vi "Test Interpolation.vi"() -> ()   [LabVIEW 2012]
doc: "This example shows the operation of the 1D interpolation VI using three selectable test sets."
uses:
  <vilib>/gmath/NI_Gmath.lvlib
panel:
  in  "stop":bool
  in  "Tab Control":enum32{"Graph", "Data"}(tab)
  out "1D Interpolation Graph":cluster{"yi":dbl[], "ramp data":dbl[]}[](graph)
  out "Interpolated Data":dbl[][](array[numeric])
  out "Original Data":dbl[][](array[numeric])
  in  "Method":i32(ring)=2 items=["nearest", "linear", "spline", "cubic Hermite", "Lagrange"]
  in  "Data Sets":enum16{"Test Set 1", "Test Set 2", "Test Set 3"}(ring)
  # "The following example shows the operation of the 1D interpolation VI using three selectable test sets.\n\nInstructions:\n1) Run the VI\n2) Modify the Data Sets and interpolation Method, and view the results on both the Graph and Data tabs\n3) Stop the VI and look at the Block Diagram for more information"
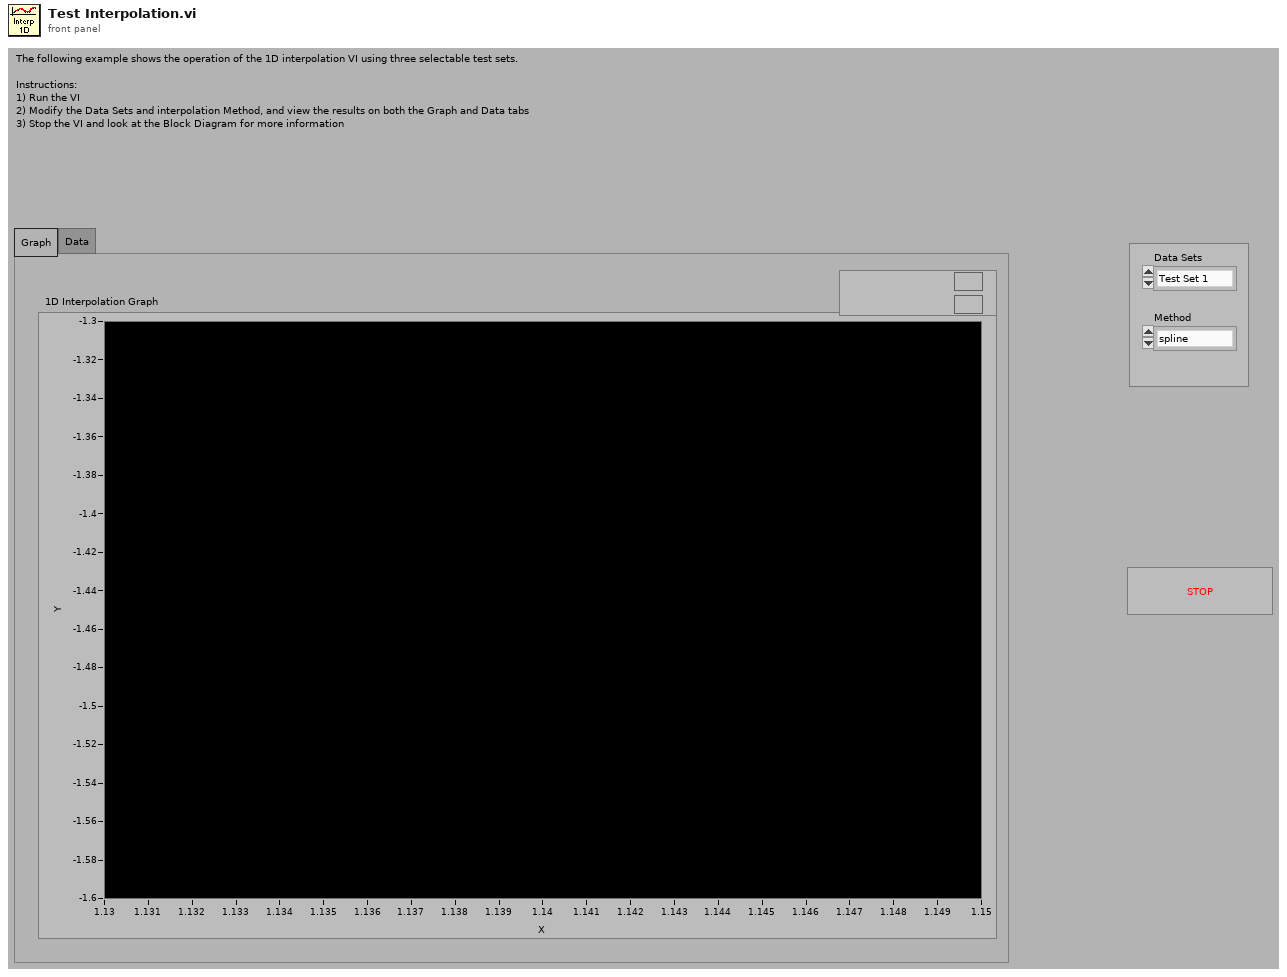
[diagram p1: front panel]
types:
  T1 = cluster{"starting value":dbl, "increment":dbl, "final value":dbl}
  T2 = cluster{"Fluke Voltage":dbl[], "Magnetic Field":dbl[]}
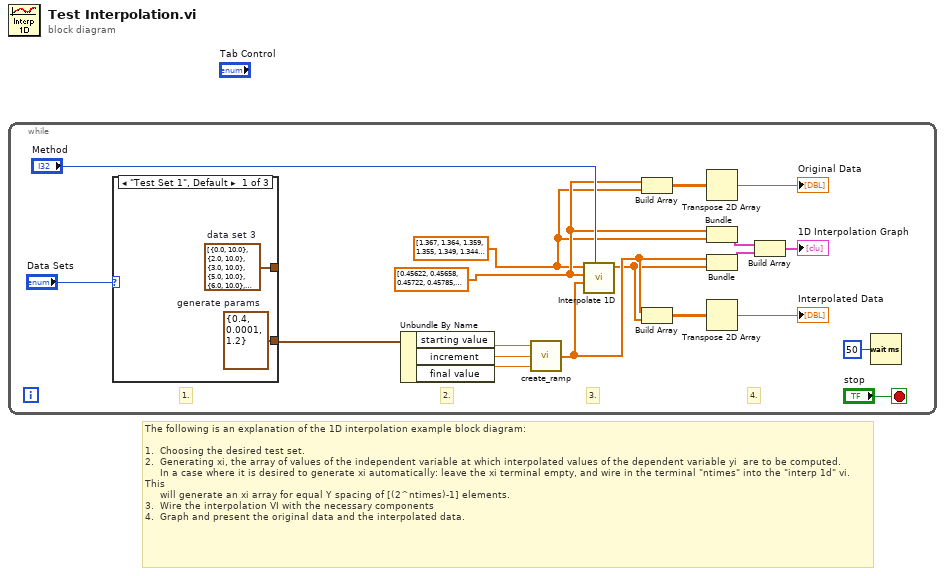
[diagram p0: block diagram]
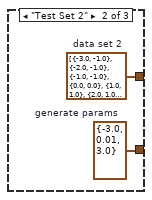
[diagram p2: hidden frame]
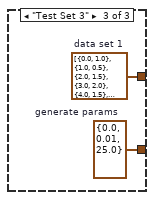
[diagram p3: hidden frame]
diagram:
  # "The following is an explanation of the 1D interpolation example block diagram:\n\n1.  Choosing the desired test set.\n2.  Generating xi, the array of values of the independent variable at which interpolated values of the dependent variable yi  are to be computed. \n     In a case where it is desired to generate xi automatically: leave the xi terminal empty, and wire in the terminal \"ntimes\" into the \"interp 1d\" vi.  This\n     will generate an xi array for equal Y spacing of [(2^ntimes)-1] elements.\n3.  Wire the interpolation VI with the necessary components\n4.  Graph and present the original data and the interpolated data."
  n1 = while {
    stop <- "stop" stop-if-true
    w1 = dbl[] [1.367, 1.364, 1.359, 1.355, 1.349, 1.344, 1.339, 1.333, 1.328, 1.322, 1.317, 1.31, 1.304, 1.297, 1.291, 1.284, 1.277, 1.269, 1.261, 1.253, 1.245, 1.236, 1.227, 1.218, 1.209, 1.1985, 1.188, 1.178, 1.166, 1.1545, 1.143, 1.131, 1.118, 1.105, 1.091, 1.077, 1.062, 1.046, 1.03, 1.013, 1.001, 0.988, 0.975, 0.961, 0.947, 0.935, 0.924, 0.912, 0.899, 0.887, 0.874, 0.86, 0.847, 0.833, 0.818, 0.804, 0.79, 0.7795, 0.769, 0.759, 0.749, 0.739, 0.7285, 0.717, 0.707, 0.697, 0.687, 0.676, 0.6656, 0.655, 0.644, 0.633, 0.623, 0.6125, 0.602, 0.5915, 0.581, 0.57, 0.56, 0.549, 0.538, 0.527, 0.516, 0.507, 0.496, 0.486, 0.475, 0.464, 0.454, 0.443, 0.432, 0.421, 0.411, 0.4, 0.388, 0.377, 0.367, 0.355, 0.344, 0.333, 0.322, 0.312, 0.301, 0.29, 0.279, 0.267, 0.256, 0.245, 0.234, 0.223, 0.2125, 0.2015, 0.1901, 0.1788, 0.1674, 0.1568, 0.1455, 0.1342, 0.1234, 0.1128, 0.1021, 0.0907, 0.0843, 0.0795, 0.0737, 0.0684, 0.0633, 0.0569, 0.0521, 0.0461, 0.0408, 0.0348, 0.0298, 0.0241, 0.01869, 0.01222, -0.00055, -0.00546, -0.0101, -0.01606, -0.02117, -0.02672, -0.032, -0.03775, -0.0428, -0.0482, -0.0539, -0.059, -0.0649, -0.0762, -0.0871, -0.0975, -0.1082, -0.1192, -0.1304, -0.1414, -0.1524, -0.1635, -0.1746, -0.1855, -0.1956, -0.2066, -0.2179, -0.2285, -0.2394, -0.2507, -0.2614, -0.2724, -0.284, -0.294, -0.305, -0.316, -0.327, -0.337, -0.348, -0.359, -0.37, -0.381, -0.391, -0.402, -0.412, -0.423, -0.434, -0.4445, -0.456, -0.465, -0.476, -0.486, -0.4965, -0.507, -0.518, -0.528, -0.539, -0.549, -0.56, -0.57, -0.581, -0.591, -0.601, -0.6115, -0.622, -0.632, -0.6425, -0.653, -0.663, -0.673, -0.682, -0.693, -0.704, -0.715, -0.724, -0.744, -0.755, -0.765, -0.774, -0.783, -0.793, -0.803, -0.812, -0.822, -0.831, -0.84, -0.849, -0.858, -0.867, -0.876, -0.884, -0.892, -0.9, -0.908, -0.9165, -0.928, -0.94, -0.951, -0.961, -0.971, -0.982, -0.992, -1.0, -1.01, -1.019, -1.028, -1.037, -1.045, -1.053, -1.062, -1.069, -1.079, -1.089, -1.098, -1.108, -1.116, -1.125, -1.134, -1.142, -1.151, -1.159, -1.167, -1.174, -1.182, -1.189, -1.2, -1.21, -1.22, -1.229, -1.238, -1.247, -1.256, -1.264, -1.272, -1.28, -1.287, -1.294, -1.3, -1.307, -1.313, -1.319, -1.324, -1.331, -1.337, -1.342, -1.348, -1.353, -1.358, -1.358, -1.362] ("Magnetic Field")
    w2 = dbl[] [0.45622, 0.45658, 0.45722, 0.45785, 0.45847, 0.45912, 0.45978, 0.46055, 0.46125, 0.46197, 0.4627, 0.46348, 0.46431, 0.46513, 0.46599, 0.4669, 0.46789, 0.46884, 0.46989, 0.47095, 0.47211, 0.47325, 0.47445, 0.47572, 0.47704, 0.47841, 0.47983, 0.48132, 0.48288, 0.48459, 0.48629, 0.48807, 0.48994, 0.49187, 0.49392, 0.49611, 0.49843, 0.5008, 0.50341, 0.50614, 0.50807, 0.51009, 0.51218, 0.51444, 0.51669, 0.51862, 0.52042, 0.52239, 0.52451, 0.52666, 0.52885, 0.53124, 0.53363, 0.53607, 0.53868, 0.54127, 0.54383, 0.5456, 0.54747, 0.54926, 0.55115, 0.55305, 0.555, 0.55713, 0.55886, 0.56084, 0.56277, 0.56477, 0.56675, 0.56878, 0.5708, 0.57294, 0.57493, 0.57686, 0.57898, 0.58109, 0.58327, 0.58542, 0.58753, 0.58974, 0.59195, 0.59421, 0.59637, 0.59843, 0.60077, 0.6027, 0.60502, 0.60731, 0.60961, 0.61205, 0.61435, 0.61676, 0.619, 0.62144, 0.62387, 0.62635, 0.6288, 0.63128, 0.6338, 0.63639, 0.63885, 0.6412, 0.64379, 0.64643, 0.64905, 0.65165, 0.65427, 0.65688, 0.65951, 0.66212, 0.66469, 0.66743, 0.67023, 0.67292, 0.6757, 0.67842, 0.68123, 0.68401, 0.68678, 0.68943, 0.69218, 0.69515, 0.69671, 0.69793, 0.69944, 0.70081, 0.70215, 0.70377, 0.70505, 0.70659, 0.708, 0.70961, 0.71087, 0.71237, 0.71381, 0.71552, 0.7189, 0.72022, 0.72144, 0.72305, 0.72441, 0.72592, 0.72736, 0.7289, 0.73029, 0.73172, 0.73329, 0.73471, 0.73631, 0.73939, 0.74236, 0.74518, 0.74821, 0.75131, 0.75442, 0.75752, 0.76062, 0.76378, 0.76693, 0.77006, 0.77295, 0.77608, 0.77922, 0.78238, 0.78554, 0.78877, 0.79198, 0.79512, 0.79838, 0.80139, 0.8046, 0.80793, 0.81117, 0.81429, 0.81758, 0.82082, 0.82416, 0.82743, 0.83061, 0.83382, 0.83692, 0.84037, 0.84372, 0.8469, 0.85018, 0.85319, 0.85649, 0.8595, 0.86277, 0.86609, 0.86959, 0.87277, 0.87609, 0.87945, 0.88274, 0.88611, 0.88934, 0.89265, 0.89576, 0.8991, 0.90238, 0.90566, 0.90905, 0.91233, 0.91559, 0.91898, 0.92182, 0.92553, 0.92871, 0.9322, 0.93527, 0.94175, 0.945, 0.94816, 0.95121, 0.95425, 0.9574, 0.96052, 0.96369, 0.96674, 0.96981, 0.97275, 0.97578, 0.9786, 0.98149, 0.9844, 0.98712, 0.9899, 0.99266, 0.99526, 0.99796, 1.00177, 1.00548, 1.00926, 1.01271, 1.01613, 1.01958, 1.02279, 1.02587, 1.0291, 1.03204, 1.03491, 1.03779, 1.04052, 1.04322, 1.046, 1.04855, 1.05187, 1.05508, 1.05821, 1.06132, 1.06427, 1.06717, 1.06999, 1.07265, 1.0756, 1.0782, 1.08079, 1.08318, 1.08563, 1.08804, 1.09148, 1.09475, 1.09792, 1.10093, 1.10388, 1.10671, 1.10948, 1.11207, 1.11457, 1.11704, 1.11926, 1.12148, 1.12357, 1.12556, 1.12751, 1.12944, 1.13126, 1.13308, 1.13501, 1.13663, 1.13825, 1.13991, 1.14145, 1.14155, 1.1419] ("Fluke Voltage")
    # "4."
    # "3."
    # "2."
    # "1."
    n2 = case shown="\"Test Set 1\", Default" "Data Sets" {
      tunnel: [w21 w23 w25] -> _
      tunnel: [w20 w22 w24] -> w18
      frame "Test Set 1", Default {
        w20 = T1 {"starting value"=0.4, "increment"=0.0001, "final value"=1.2}  # generate params
        w21 = cluster{"x":dbl, "y":dbl}[] [{"x"=0.0, "y"=10.0}, {"x"=2.0, "y"=10.0}, {"x"=3.0, "y"=10.0}, {"x"=5.0, "y"=10.0}, {"x"=6.0, "y"=10.0}, {"x"=8.0, "y"=10.0}, {"x"=9.0, "y"=10.5}, {"x"=11.0, "y"=15.0}, {"x"=12.0, "y"=50.0}, {"x"=14.0, "y"=60.0}, {"x"=15.0, "y"=85.0}]  # data set 3
      }
      frame "Test Set 2" {
        w22 = T1 {"starting value"=-3.0, "increment"=0.01, "final value"=3.0}  # generate params
        w23 = cluster{"x":dbl, "y":dbl}[] [{"x"=-3.0, "y"=-1.0}, {"x"=-2.0, "y"=-1.0}, {"x"=-1.0, "y"=-1.0}, {"x"=0.0, "y"=0.0}, {"x"=1.0, "y"=1.0}, {"x"=2.0, "y"=1.0}, {"x"=3.0, "y"=1.0}]  # data set 2
      }
      frame "Test Set 3" {
        w24 = T1 {"starting value"=0.0, "increment"=0.01, "final value"=25.0}  # generate params
        w25 = cluster{"x":dbl, "y":dbl}[] [{"x"=0.0, "y"=1.0}, {"x"=1.0, "y"=0.5}, {"x"=2.0, "y"=1.5}, {"x"=3.0, "y"=2.0}, {"x"=4.0, "y"=1.5}, {"x"=5.0, "y"=0.5000000000000002}, {"x"=6.0, "y"=0.0}, {"x"=7.0, "y"=0.4999999999999998}, {"x"=8.0, "y"=1.4999999999999998}, {"x"=9.0, "y"=2.0}, {"x"=10.0, "y"=2.0}, {"x"=11.0, "y"=2.0}, {"x"=12.0, "y"=2.0}, {"x"=13.0, "y"=-0.5}, {"x"=14.0, "y"=-0.5}, {"x"=15.0, "y"=2.0}, {"x"=16.0, "y"=0.0}, {"x"=17.0, "y"=0.0}, {"x"=18.0, "y"=0.0}, {"x"=19.0, "y"=0.0}, {"x"=20.0, "y"=1.0}, {"x"=21.0, "y"=0.0}, {"x"=22.0, "y"=0.0}, {"x"=23.0, "y"=0.0}, {"x"=24.0, "y"=2.0}]  # data set 1
      }
    }
    n3 = Unbundle By Name(w18) -> ("starting value"=w12:dbl, "increment"=w11:dbl, "final value"=w10:dbl)
    n4 = call "create_ramp.vi"("final value"=w10, "increment"=w11, "starting value"=w12) -> ("ramp data"=w6:dbl[])
    n5 = call <vilib>:"Interpolate 1D.vi"("method"="Method", "xi"=w6, "X"=w2, "Y"=w1) -> ("yi"=w5:dbl[])  [unwired: 5 in, 2 out]
    n6 = Build Array(w2, w1) -> (w9:dbl[][])
    n7 = Build Array(w6, w5) -> (w7:dbl[][])
    n8 = Transpose 2D Array(2D array=w9) -> (transposed array=→"Original Data":dbl[][])
    n9 = Bundle("Fluke Voltage"=w2, "Magnetic Field"=w1) -> (w15:T2)  [unwired: 1 in]
    n10 = Bundle("ramp data"=w6, "yi"=w5) -> (w16:cluster{"ramp data":dbl[], "yi":dbl[]})  [unwired: 1 in]
    n11 = Transpose 2D Array(2D array=w7) -> (transposed array=→"Interpolated Data":dbl[][])
    n12 = Build Array(w15, w16) -> (→"1D Interpolation Graph":cluster{"ramp data":dbl[], "yi":dbl[]}[])
    n13 = Wait (ms)(milliseconds to wait=u32 50) -> ()  [unwired: 1 out]
  }
